vi "Write File Setup.vi"(8 "error in (no error)":errorcluster, 10 "Setup":T1, 11 "Setup File in":refnum<class "Setup File.lvclass">) -> (0 "error out":errorcluster, 3 "Setup File out":refnum<class "Setup File.lvclass">)   [LabVIEW 2018, in "Setup File.lvclass"]
doc: "Este VI escreve na classe a configuração contida no cluster \"Setup\"."
uses:
  Setup File.lvclass
  Setup File.lvclass/Setup File.ctl
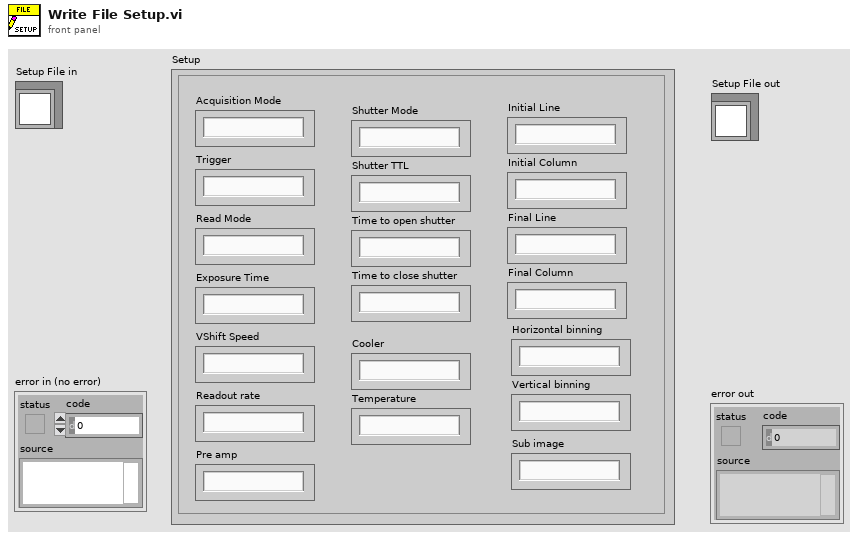
[diagram p1: front panel]
types:
  T1 = cluster{"Read Mode":string, "Acquisition Mode":string, "Trigger":string, "Exposure Time":string, "VShift Speed":string, "Readout rate":string, "Pre amp":string, "Shutter Mode":string, "Shutter TTL":string, "Time to open shutter":string, "Time to close shutter":string, "Cooler":string, "Temperature":string, "Initial Line":string, "Initial Column":string, "Final Line":string, "Final Column":string, "Horizontal binning":string, "Vertical binning":string, "Sub image":string}
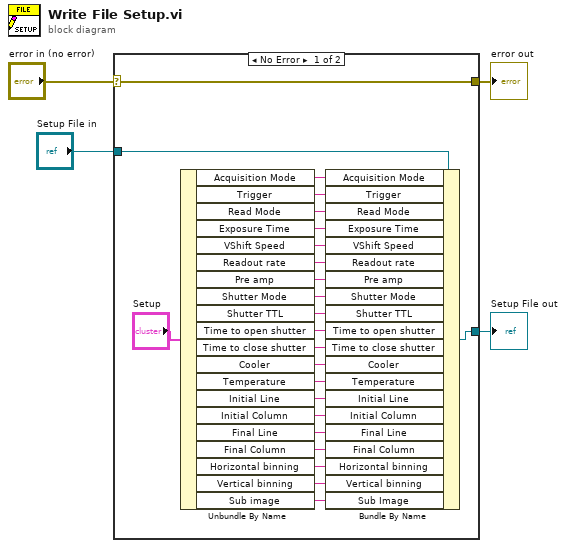
[diagram p0: block diagram]
diagram:
  n1 = case shown="No Error" "error in (no error)" {
    selector: "error in (no error)" -> [w28 w29]
    tunnel: [w28 w29] -> w3
    tunnel: [w26 w30] -> w1
    tunnel: "Setup File in" -> [w27 w30]
    frame No Error {
      n2 = Unbundle By Name("Setup") -> ("Acquisition Mode"=w6:string, "Trigger"=w7:string, "Read Mode"=w8:string, "Exposure Time"=w9:string, "VShift Speed"=w10:string, "Readout rate"=w11:string, "Pre amp"=w12:string, "Shutter Mode"=w13:string, "Shutter TTL"=w14:string, "Time to open shutter"=w15:string, "Time to close shutter"=w16:string, "Cooler"=w17:string, "Temperature"=w18:string, "Initial Line"=w19:string, "Initial Column"=w20:string, "Final Line"=w21:string, "Final Column"=w22:string, "Horizontal binning"=w23:string, "Vertical binning"=w24:string, "Sub image"=w5:string)
      n3 = Bundle By Name(cluster=w27, "Acquisition Mode"=w6, "Trigger"=w7, "Read Mode"=w8, "Exposure Time"=w9, "VShift Speed"=w10, "Readout rate"=w11, "Pre amp"=w12, "Shutter Mode"=w13, "Shutter TTL"=w14, "Time to open shutter"=w15, "Time to close shutter"=w16, "Cooler"=w17, "Temperature"=w18, "Initial Line"=w19, "Initial Column"=w20, "Final Line"=w21, "Final Column"=w22, "Horizontal binning"=w23, "Vertical binning"=w24, "Sub Image"=w5) -> (w26:refnum<class "Setup File.lvclass">)
    }
    frame Error {
    }
  }
  "error out" <- w3
  "Setup File out" <- w1
